vi "datachopper.vi"(6 "xmax":dbl=40.0, 8 "xmin":dbl=-40.0, 9 "ymin":dbl, 10 "ymax":dbl=40.0, 11 "input":dbl[][](array[numeric])) -> (0 "h_ave":dbl, 1 "y_ave":dbl, 2 "x_ave":dbl, 3 "output":dbl[][](array[numeric]))   [LabVIEW 2012]
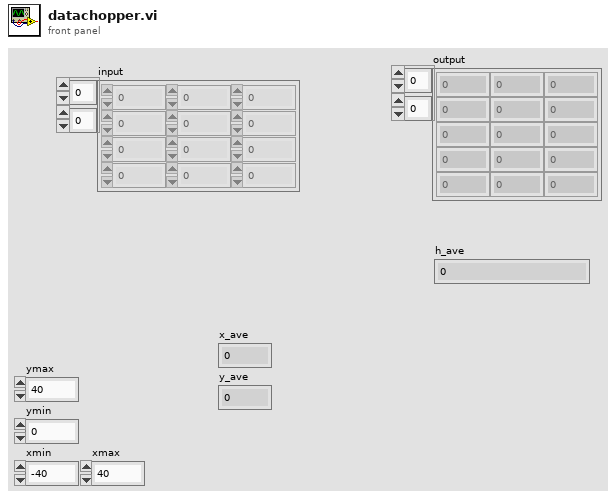
[diagram p1: front panel]
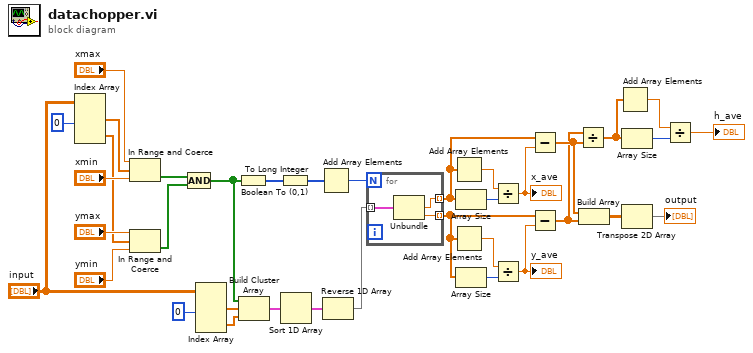
[diagram p0: block diagram]
diagram:
  n1 = Index Array(array="input", index (col) #1=0 ("disabled index (col)")) -> (element #1=w33:dbl[], element #2=w28:dbl[])  [unwired: 3 in]
  n2 = In Range and Coerce(upper limit="xmax", x=w33, lower limit="xmin") -> (In Range?=w27:bool[])  [unwired: 1 out]
  n3 = In Range and Coerce(upper limit="ymax", x=w28, lower limit="ymin") -> (In Range?=w26:bool[])  [unwired: 1 out]
  n4 = Compound Arithmetic op=AND(w27, w26) -> (w15:bool[])
  n5 = Index Array(array="input", index (col) #1=0 ("disabled index (col)")) -> (element #1=w17:dbl[], element #2=w16:dbl[])  [unwired: 3 in]
  n6 = Boolean To (0,1)(Boolean=w15) -> (0, 1=w21:i16[])
  n7 = Build Cluster Array(w15, w17, w16) -> (w19:cluster{bool, "element":dbl, "element":dbl}[])
  n8 = To Long Integer(number=w21) -> (32bit integer=w22:i32[])
  n9 = Sort 1D Array(array=w19) -> (sorted array=w20:cluster{bool, "element":dbl, "element":dbl}[])
  n10 = Add Array Elements(numeric array=w22) -> (sum=w23:i32)
  n11 = Reverse 1D Array(array=w20) -> (reversed array=w24:cluster{bool, "element":dbl, "element":dbl}[])
  n12 = for {
    N: w23 -> [_]
    tunnel: w24 -> [w39] mode=indexing
    tunnel: [w38] -> w11 mode=indexing
    tunnel: [w37] -> w7 mode=indexing
    n13 = Unbundle(w39) -> ("element"=w38:dbl, "element"=w37:dbl)  [unwired: 1 out]
  }
  n14 = Add Array Elements(numeric array=w11) -> (sum=w14:dbl)
  n15 = Add Array Elements(numeric array=w7) -> (sum=w8:dbl)
  n16 = Array Size(array=w11) -> (size(s)=w13:i32)
  n17 = Array Size(array=w7) -> (size(s)=w9:i32)
  n18 = Divide(x=w14, y=w13) -> (x/y=w12:dbl)
  "x_ave" <- w12
  n19 = Divide(x=w8, y=w9) -> (x/y=w10:dbl)
  "y_ave" <- w10
  n20 = Subtract(x=w11, y=w12) -> (x-y=w6:dbl[])
  n21 = Subtract(x=w7, y=w10) -> (x-y=w5:dbl[])
  n22 = Divide(x=w5, y=w6) -> (x/y=w2:dbl[])
  n23 = Build Array(w6, w5) -> (w25:dbl[][])
  n24 = Add Array Elements(numeric array=w2) -> (sum=w3:dbl)
  n25 = Array Size(array=w2) -> (size(s)=w4:i32)
  n26 = Transpose 2D Array(2D array=w25) -> (transposed array=→"output":dbl[][])
  n27 = Divide(x=w3, y=w4) -> (x/y=→"h_ave":dbl)
